vi "create server listener.vi"(8 "error in":errorcluster) -> (0 "error out":errorcluster, 3 "lvlibretls server listener out":refnum<class "lvlibretls server listener.lvclass">)   [LabVIEW 2016, in "lvlibretls server listener.lvclass"]
doc: "Creates a server context, which includes a parent configuration context. When accept is called, the server context is reconfigured with the config context before creating the socket context."
uses:
  lvlibretls server listener.lvclass
  C:/Users/IEUser/Desktop/tlssimple/libretls/context parent/lvlibretls configurable context.lvclass
  lvlibretls server listener.lvclass/lvlibretls server listener.ctl
  context parent/lvlibretls configurable context.lvclass
  lv tls dll.lvlib
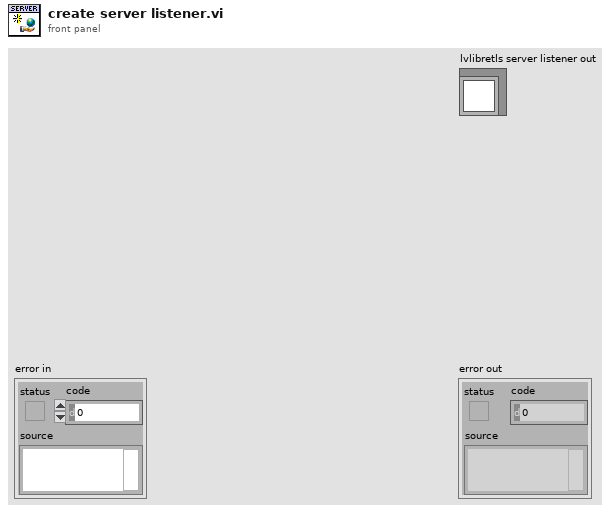
[diagram p1: front panel]
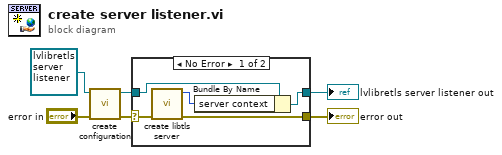
[diagram p0: block diagram]
diagram:
  n1 = call "create configuration.vi"("error in"="error in", "lvlibretls configurable context in"=refnum<class "lvlibretls server listener.lvclass"> refnum ("lvlibretls server listener in")) -> ("error out"=w2:errorcluster, "lvlibretls configurable context out"=w5:refnum<class "lvlibretls server listener.lvclass">)  [unwired: 8 in]
  n2 = case shown="No Error" w2 {
    selector: w2 -> [w9 w13]
    tunnel: w5 -> [w11 w12]
    tunnel: [w10 w12] -> w4
    tunnel: [w8 w13] -> w1
    frame No Error {
      n3 = call "create libtls server.vi"("error in"=w9) -> ("error out"=w8:errorcluster, "server out"=w7:u64)  [unwired: 9 in]
      n4 = Bundle By Name(cluster=w11, "server context"=w7) -> (w10:refnum<class "lvlibretls server listener.lvclass">)
    }
    frame Error {
    }
  }
  "error out" <- w1
  "lvlibretls server listener out" <- w4
